vi "Configure Multi Eval Meas Trigger Timeout.vi"(7 "Measurement Trigger Timeout (0.1)":dbl=0.1 format="%^.3e", 8 "error in (no error)":errorcluster, 9 "Trigger Timeout Enabled (Off)":bool, 10 "Instance (1)":T1=1, 11 "VISA resource name":refnum<visa-resource-name>) -> (0 "error out":errorcluster, 3 "VISA resource name out":refnum<visa-resource-name>)   [LabVIEW 2020, in "Rohde&Schwarz CMWXP NR FR1 Measurement.lvlib"]
doc: "Selects the maximum time that the measurement waits for a trigger event before it stops in remote control mode or indicates a trigger timeout in manual operation mode. This setting has no influence on Free Run measurements.\n\nAttributes:\nRSCMWXPNRFR1M_ATTR_MULTI_EVAL_MEAS_TRIGGER_TIMEOUT_ENABLED\nRSCMWXPNRFR1M_ATTR_MULTI_EVAL_MEAS_TRIGGER_TIMEOUT\n\nRemote-control command:\nTRIGger:NRSub:MEAS<i>:MEValuation:TOUT"
uses:
  <instrlib>/Rohde&Schwarz CMWXP NR FR1 Measurement/Rohde&Schwarz CMWXP NR FR1 Measurement.lvlib
  <instrlib>/Rohde&Schwarz CMWXP NR FR1 Measurement/Private/_Instance.ctl
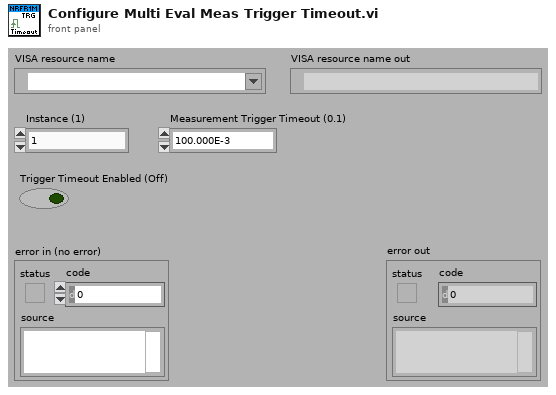
[diagram p1: front panel]
types:
  T1 = typedef "Rohde&Schwarz CMWXP NR FR1 Measurement.lvlib/_Instance.ctl" = i32
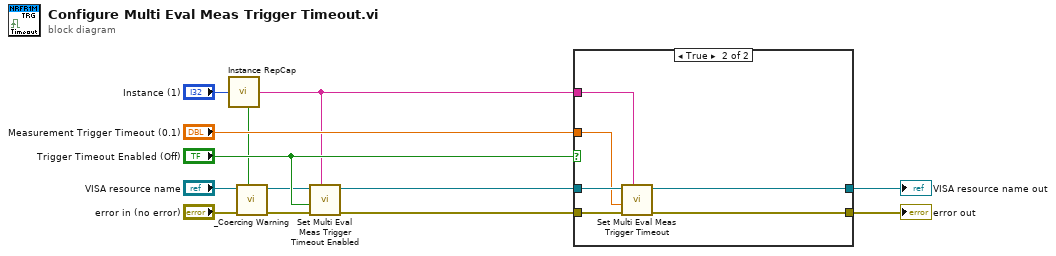
[diagram p0: block diagram]
diagram:
  n1 = call <instrlib>:"Instance RepCap.vi"("Instance In"="Instance (1)") -> ("In Range?"=w1:bool, "RepCap Identifier Out"=w6:string)  [unwired: 1 in]
  n2 = call <instrlib>:"_Coercing Warning.vi"("In Range?"=w1, "error in (no error)"="error in (no error)", "VISA resource name"="VISA resource name") -> ("error out"=w3:errorcluster, "VISA resource name out"=w2:refnum<visa-resource-name>)  [unwired: 7 in]
  n3 = call "Set Multi Eval Meas Trigger Timeout Enabled"("Repeated Capabilities"=w6, "error in (no error)"=w3, "Multi Eval Meas Trigger Timeout Enabled (OFF)"="Trigger Timeout Enabled (Off)", "instrument handle"=w2) -> ("error out"=w10:errorcluster, "instrument handle out"=w11:refnum<visa-resource-name>)  [unwired: 6 in]
  n4 = case shown="True" "Trigger Timeout Enabled (Off)" {
    tunnel: [w14 w21] -> w13
    tunnel: [w15 w20] -> w12
    tunnel: w11 -> [w15 w19]
    tunnel: w10 -> [w14 w18]
    tunnel: "Measurement Trigger Timeout (0.1)" -> [_ w17]
    tunnel: w6 -> [_ w16]
    frame False {
    }
    frame True {
      n5 = call "Set Multi Eval Meas Trigger Timeout"("Repeated Capabilities"=w16, "error in (no error)"=w18, "Multi Eval Meas Trigger Timeout (0.0)"=w17, "instrument handle"=w19) -> ("error out"=w21:errorcluster, "instrument handle out"=w20:refnum<visa-resource-name>)  [unwired: 6 in]
    }
  }
  "error out" <- w13
  "VISA resource name out" <- w12
